vi "XGT 개별쓰기 응답프레임.vi"() -> ()   [LabVIEW 2012]
panel:
  out "에러코드":string
  out "Tail":string
  out "명령어 타입":string="SS"
  out "국번과 명령어":string="01W"
  out "Header":string
  in  "응답프레임":string="\u000601WSS\u0003"
  # "ACK응답 예: 0630 3157 5353 03"
  # "NAK응답 예: 1530 3157 5353 3030 3030 03"
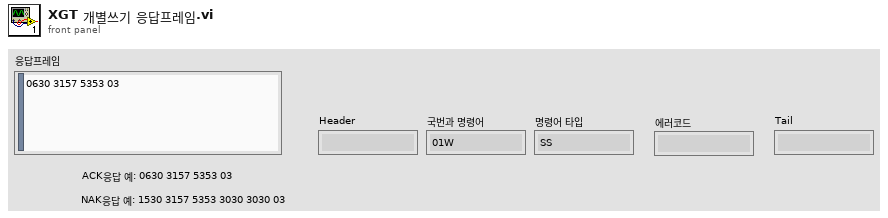
[diagram p1: front panel]
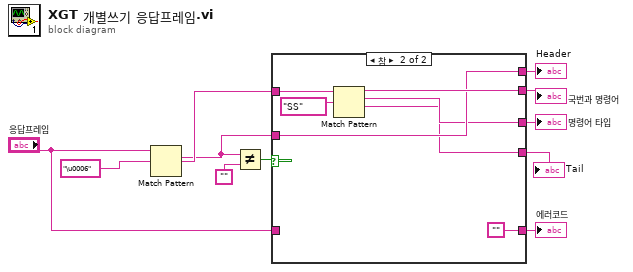
[diagram p0: block diagram]
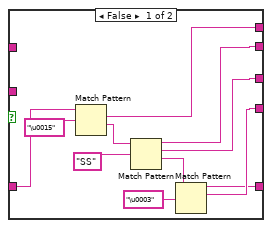
[diagram p2: hidden frame]
diagram:
  n1 = Match Pattern(string="응답프레임", regular expression="\u0006" ("정규식")) -> (match substring=w7:string, after substring=w8:string)  [unwired: 1 in, 2 out]
  n2 = Not Equal?(x=w7, y="") -> (x != y?=w9:bool)
  n3 = case shown="참" w9 {
    tunnel: w8 -> [_ w28]
    tunnel: w7 -> [_ w26]
    tunnel: [w16 w27] -> w5
    tunnel: [w20 w26] -> w6
    tunnel: [w17 w25] -> w4
    tunnel: [w13 w24] -> w3
    tunnel: "응답프레임" -> [w22 _]
    tunnel: [w12 ""] -> w1
    frame False {
      n4 = Match Pattern(string=w22, regular expression="\u0015" ("정규식")) -> (match substring=w20:string, after substring=w19:string)  [unwired: 1 in, 2 out]
      n5 = Match Pattern(string=w19, regular expression="SS" ("정규식")) -> (before substring=w16:string, match substring=w17:string, after substring=w15:string)  [unwired: 1 in, 1 out]
      n6 = Match Pattern(string=w15, regular expression="\u0003" ("정규식")) -> (before substring=w12:string, match substring=w13:string)  [unwired: 1 in, 2 out]
    }
    frame True {
      n7 = Match Pattern(string=w28, regular expression="SS" ("정규식")) -> (before substring=w27:string, match substring=w25:string, after substring=w24:string)  [unwired: 1 in, 1 out]
    }
  }
  "Header" <- w6
  "국번과 명령어" <- w5
  "명령어 타입" <- w4
  "Tail" <- w3
  "에러코드" <- w1
